vi "uBroker_Fanout.vi"(9 "uMsg":refnum<class "uMsg.lvclass">, 10 "uPub":refnum<class "uClient_Publisher.lvclass">, 11 "Cluster in":T2) -> (3 "Cluster out":T2)   [LabVIEW 2021, in "uFramework.lvlib" / "uBroker.lvclass"]
uses:
  uBroker.lvclass
  TypeDef_uBrokerTopic.ctl
  uMsg/uMsg.lvclass
  uClient_Publisher/uClient_Publisher.lvclass
  uSubscription/uSubscription.lvclass
  uClient_Subscriber/uClient_Subscriber.lvclass
  U:/Projects/uFramework/Src/uFramework/uClient/uClient.lvclass
  uMsg/uMsg.lvclass/uMsg.ctl
  <vilib>/Utility/miscctls.llb/LVMapReplaceAction.ctl
  uClient/uClient.lvclass/uClient.ctl
  uClient_Subscriber/uClient_Subscriber.lvclass/uClient_Subscriber.ctl
  uPolicy/uPolicy.lvclass/uPolicy.ctl
  uSubscription/uSubscription.lvclass/uSubscription.ctl
  uNotifyMode/uNotifyMode.lvclass/uNotifyMode.ctl
  uTransport_uActor/uTransport_uActor.lvclass/uTransport_uActor.ctl
  uTransport_Event/uTransport_Event.lvclass/uTransport_Event.ctl
  uTransport_Queue/uTransport_Queue.lvclass/uTransport_Queue.ctl
  uMsg/uMsg Rename CMD.vi
  uNotifyMode/uNotify Update.vi
  uClient/uClient_GetTransport.vi
  uClient_Subscriber/uSubscriber Get uPolicy.vi
  uPolicy/Read uNotifyMode.vi
  uPolicy/Read uStringManipulation.vi
  uTransport/uTransport_SendMsg.vi
  uTransport_uActor/uTransport_uActor_SendMsg.vi
  uTransport_Event/uTransport_Event_SendMsg.vi
  uTransport_Queue/uTransport_Queue_SendMsg.vi
  uMsg/uMsg Update Timestamp.vi
  uNotifyMode/uNotifyMode.lvclass
  uTransport/uTransport.lvclass
  uPolicy/uPolicy.lvclass
  Bin/uStringManipulation.lvlibp/uStringManipulation.lvclass
  uTransport_uActor/uTransport_uActor.lvclass
  uTransport_Event/uTransport_Event.lvclass
  uTransport_Queue/uTransport_Queue.lvclass
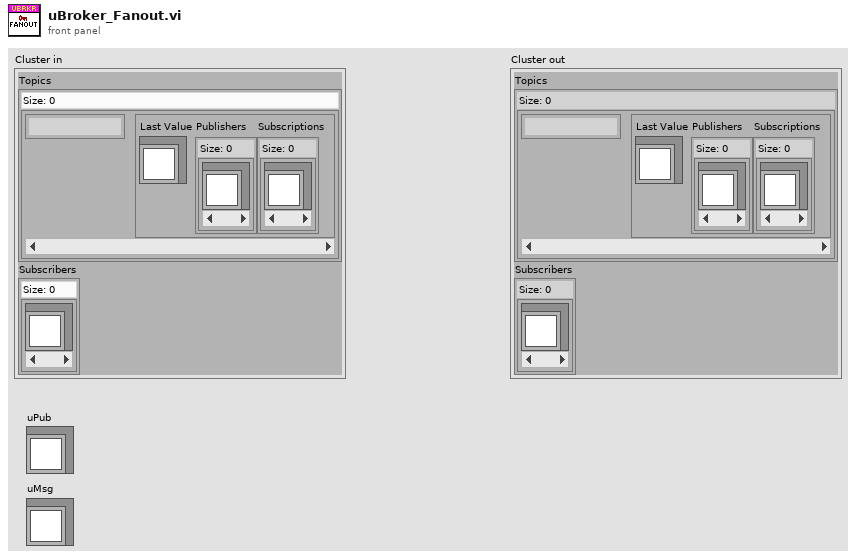
[diagram p1: front panel]
types:
  T1 = typedef "uFramework.lvlib/uBroker.lvclass/TypeDef_uBrokerTopic.ctl" = cluster{"Last Value":refnum<class "uMsg.lvclass">, "Publishers":set{refnum<class "uClient_Publisher.lvclass">}, "Subscriptions":set{refnum<class "uSubscription.lvclass">}}
  T2 = cluster{"Topics":map{string, T1}, "Subscribers":set{refnum<class "uClient_Subscriber.lvclass">}}
  T3 = typedef "LVMapReplaceAction.ctl" = enum32{"Modify Entry only if found", "Add or Modify Entry", "Delete Entry"}
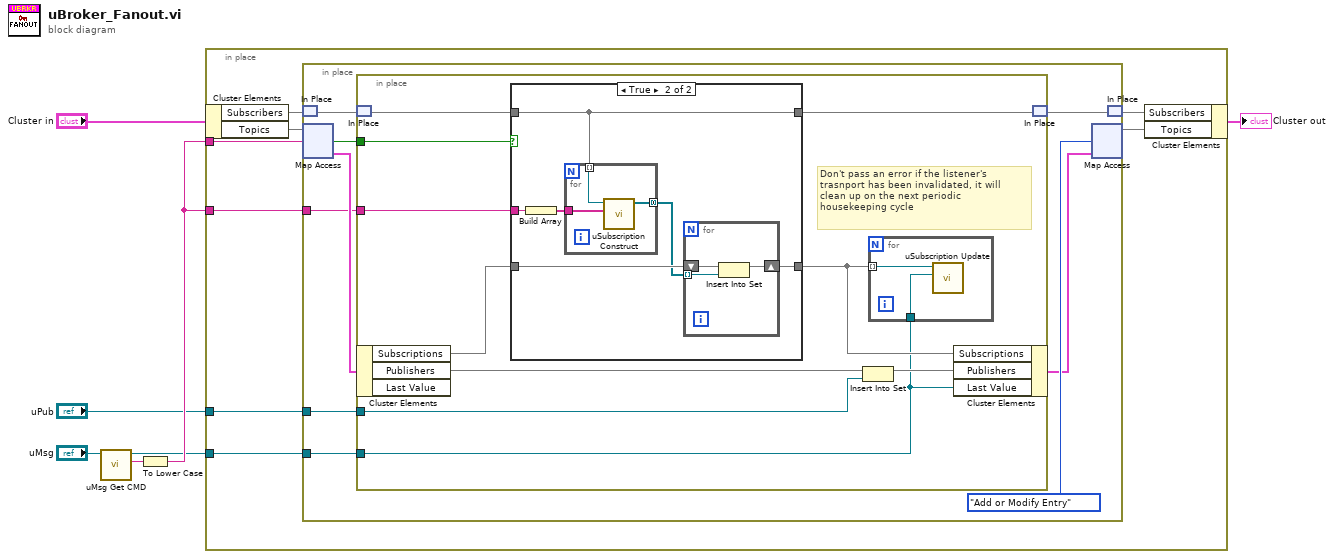
[diagram p0: block diagram]
diagram:
  n1 = call "uMsg Get CMD.vi"("uMsg in"="uMsg") -> ("CMD"=w2:string, "uMsg out"=w3:refnum<class "uMsg.lvclass">)  [unwired: 8 in, 1 out]
  n2 = To Lower Case(string=w2) -> (all lower case string=w4:string)
  n3 = in-place {
    in-place-border: w4 -> [w12]
    in-place-border: w3 -> [w13]
    in-place-border: "uPub" -> [w11]
    in-place-border: w4 -> [w10]
    n4 = in-place-cluster #1("Cluster in") -> ("Subscribers"=w9:set{refnum<class "uClient_Subscriber.lvclass">}, "Topics"=w15:map{string, T1})
    n5 = in-place {
      in-place-border: w13 -> [w23]
      in-place-border: w11 -> [w22]
      in-place-border: w10 -> [w18]
      n6 = in-place-match #2(w9) -> (w16:set{refnum<class "uClient_Subscriber.lvclass">})
      n7 = in-place-map #3(w15, w12) -> (w20:T1, w21:bool)  [unwired: 1 in]
      n8 = in-place {
        in-place-border: w23 -> [w25]
        in-place-border: w22 -> [w30]
        in-place-border: w21 -> [w34]
        in-place-border: w18 -> [w29]
        # "Don't pass an error if the listener's trasnport has been invalidated, it will clean up on the next periodic housekeeping cycle"
        n9 = in-place-match #4(w16) -> (w27:set{refnum<class "uClient_Subscriber.lvclass">})
        n10 = in-place-cluster #5(w20) -> ("Subscriptions"=w32:set{refnum<class "uSubscription.lvclass">}, "Publishers"=w28:set{refnum<class "uClient_Publisher.lvclass">})  [unwired: 1 out]
        n11 = case shown="True" w34 {
          tunnel: [w36 w42] -> w31
          tunnel: w32 -> [w36 w39]
          tunnel: w29 -> [_ w41]
          tunnel: w27 -> [w35 w37]
          tunnel: [w35 w37] -> w26
          frame False {
          }
          frame True {
            n12 = Build Array(w41) -> (w40:string[])
            n13 = for {
              tunnel: [w45] -> w38 mode=concatenating
              tunnel: w40 -> [w44]
              tunnel: w37 -> [w43] mode=indexing
              n14 = call "uSubscription Construct.vi"("Topics"=w44, "uClient_Subscriber"=w43) -> ("uSubscriptions out"=w45:refnum<class "uSubscription.lvclass">[])  [unwired: 7 in, 2 out]
            }
            n15 = for {
              shift-right: [w48] -> w42
              shift-left: w39 -> [w47]
              tunnel: w38 -> [w46] mode=indexing
              n16 = Insert Into Set(10:w46, 11:w47) -> (3:w48:set{refnum<class "uSubscription.lvclass">})  [unwired: 1 out]
            }
          }
        }
        n17 = Insert Into Set(10:w30, 11:w28) -> (3:w33:set{refnum<class "uClient_Publisher.lvclass">})  [unwired: 1 out]
        n18 = for {
          tunnel: w31 -> [w50] mode=indexing
          tunnel: w25 -> [w49]
          n19 = call "uSubscription Update.vi"("uMsg"=w49, "uSubscription in"=w50) -> ()  [unwired: 9 in, 1 out]
        }
        n20 = in-place-cluster #5("Subscriptions"=w31, "Publishers"=w33, "Last Value"=w25) -> (w19:T1)
        n21 = in-place-match #4(w26) -> (w17:set{refnum<class "uClient_Subscriber.lvclass">})
      }
      n22 = in-place-map #3(w19, LVMapReplaceAction."Add or Modify Entry" ("action")) -> (w14:map{string, T1})  [unwired: 2 out]
      n23 = in-place-match #2(w17) -> (w8:set{refnum<class "uClient_Subscriber.lvclass">})
    }
    n24 = in-place-cluster #1("Subscribers"=w8, "Topics"=w14) -> (→"Cluster out":T2)
  }
